vi "TestNumberAssumption.vi"() -> ()   [LabVIEW 2019]
panel:
  out "double precision float 2":dbl
  out "double precision float":dbl
  out "single precision float":sgl
  out "Double Along The Way":u32
  out "Single Along The Way":u32
  in  "U32":u32
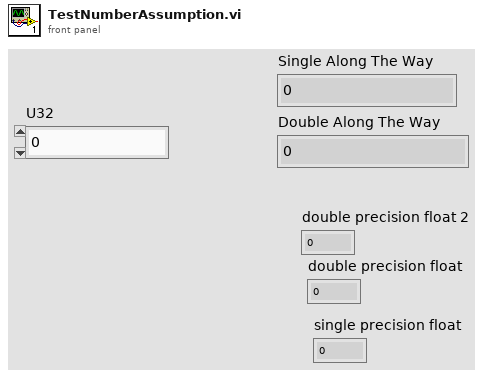
[diagram p1: front panel]
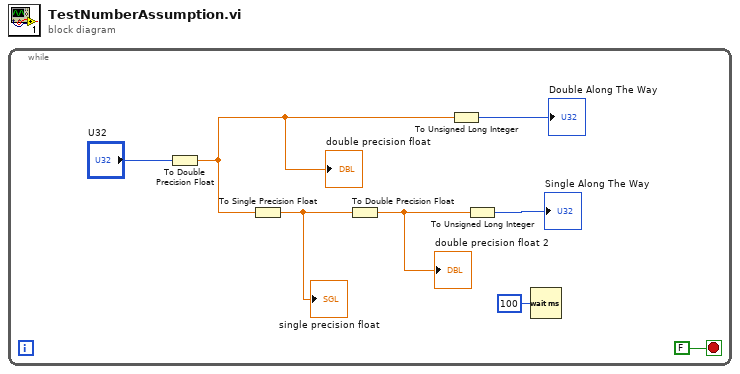
[diagram p0: block diagram]
diagram:
  n1 = while {
    stop <- FALSE stop-if-true
    n2 = To Double Precision Float(number="U32") -> (double precision float=w7:dbl)
    "double precision float" <- w7
    n3 = To Single Precision Float(number=w7) -> (single precision float=w6:sgl)
    "single precision float" <- w6
    n4 = To Double Precision Float(number=w6) -> (double precision float=w5:dbl)
    "double precision float 2" <- w5
    n5 = To Unsigned Long Integer(number=w7) -> (unsigned 32bit integer=→"Double Along The Way":u32)
    n6 = To Unsigned Long Integer(number=w5) -> (unsigned 32bit integer=→"Single Along The Way":u32)
    n7 = Wait (ms)(milliseconds to wait=u32 100) -> ()  [unwired: 1 out]
  }
